vi "Interfacetest.vi"(8 "error in (no error)":errorcluster caption="Fehler (Eingang, kein Fehler)", 11 "Device ID":T1(ring)) -> (0 "error out":errorcluster caption="Fehler (Ausgang)", 3 "Device ID Out":T1(ring))   [LabVIEW 2010]
uses:
  sub VIs v Hauptprogramm/globale Variable 1.vi
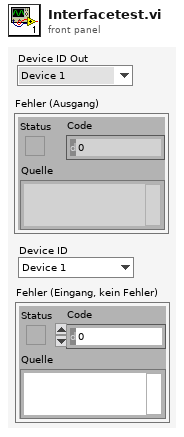
[diagram p1: front panel]
types:
  T1 = enum16{"Device 1", "Device 2", "Device 3", "Device 4", "Device 5", "Device 6", "Device 7", "Device 8"}
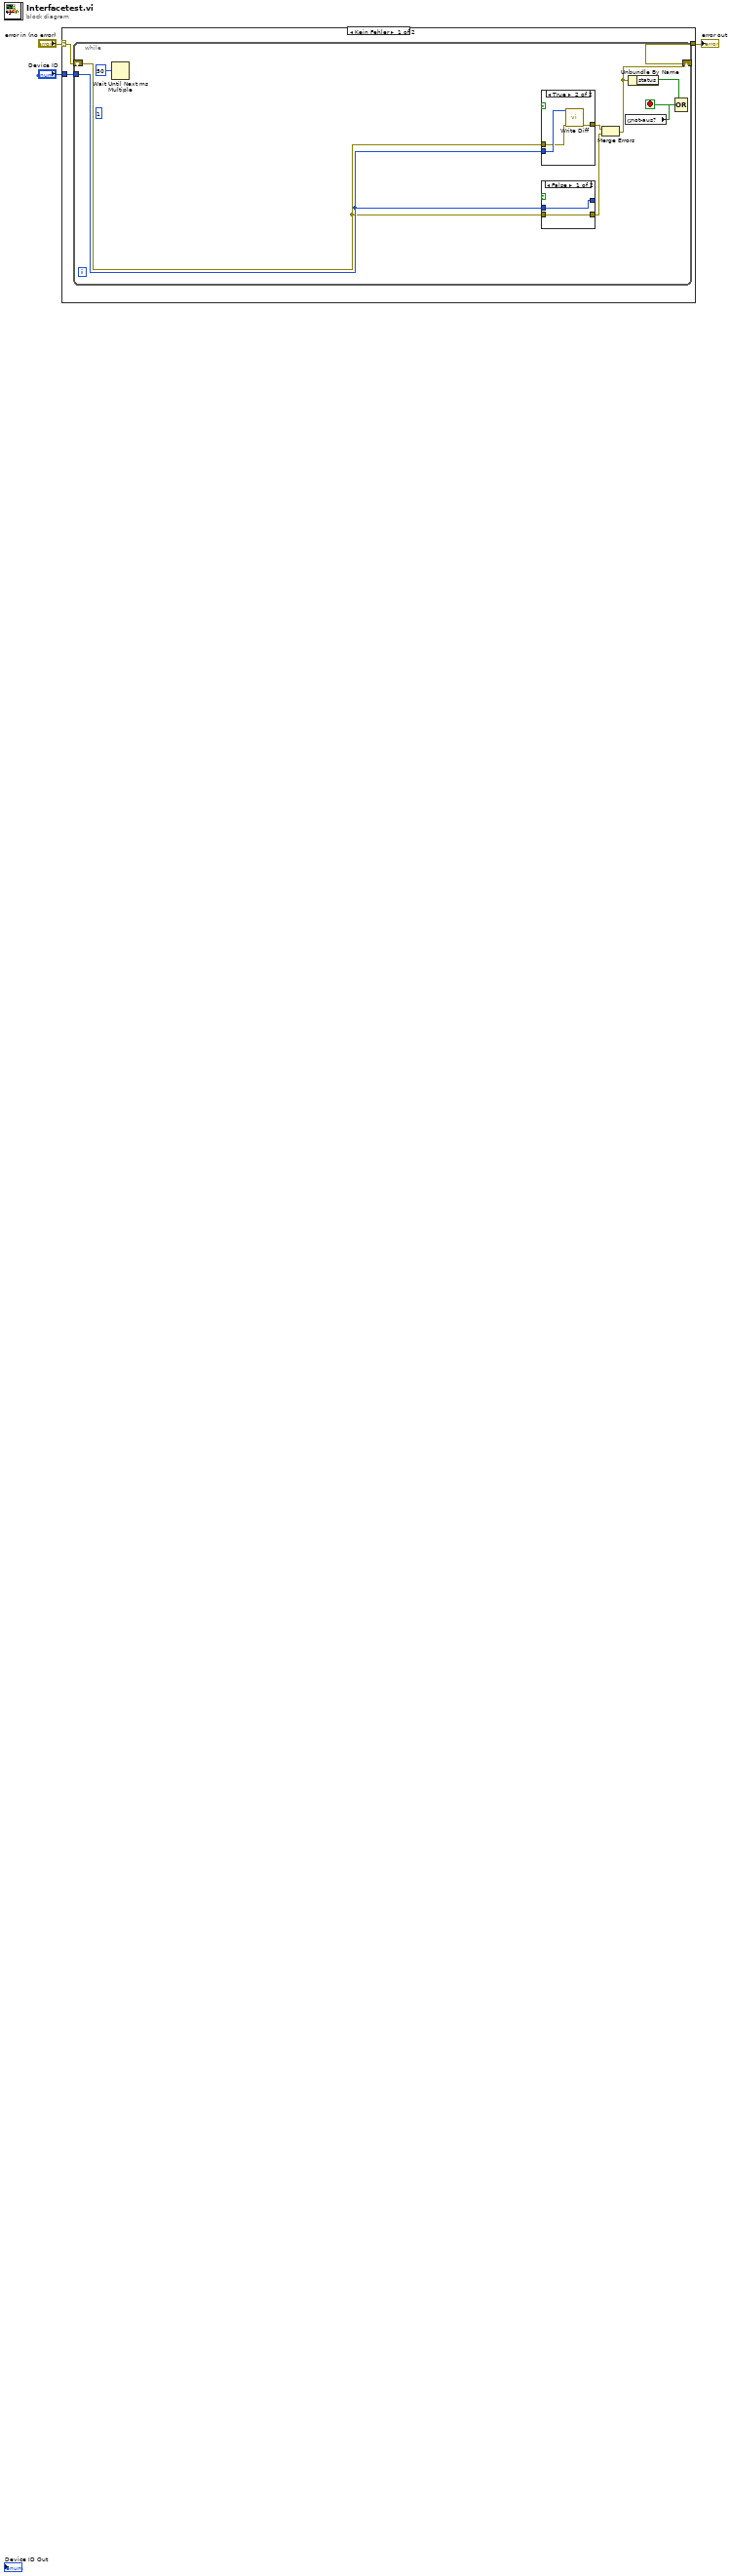
[diagram p0: block diagram]
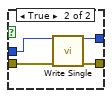
[diagram p3: hidden frame]
diagram:
  n1 = case shown="Kein Fehler" "error in (no error)" {
    selector: "error in (no error)" -> [w5 w26]
    tunnel: [w4 w26] -> w2
    tunnel: "Device ID" -> [w6 _]
    frame No Error {
      n2 = while {
        tunnel: w6 -> [w14]
        shift-right: [w10] -> w4
        shift-left: w5 -> [w11]
        stop <- w7 stop-if-true
        (unwired) 1
        n3 = Wait Until Next ms Multiple(millisecond multiple=50) -> ()  [unwired: 1 out]
        n4 = case shown="True" {
          selector: _ -> [_ _]
          tunnel: w14 -> [_ w19]
          tunnel: [w16 w18] -> w13
          tunnel: w11 -> [w16 w17]
          frame False {
          }
          frame True {
            n5 = call "Write Diff.vi"("Device ID"=w19, "error in"=w17) -> ("error out"=w18:errorcluster)  [unwired: 4 in, 9 out]
          }
        }
        n6 = case shown="False" {
          selector: _ -> [_ _]
          tunnel: [w21 w25] -> _
          tunnel: w14 -> [w21 w24]
          tunnel: [w20 w23] -> w12
          tunnel: w11 -> [w20 w22]
          frame False {
          }
          frame True {
            n7 = call "Write Single.vi"("Device ID"=w24, "error in"=w22) -> ("Device ID Out"=w25:T1, "error out"=w23:errorcluster)  [unwired: 4 in, 8 out]
          }
        }
        n8 = Merge Errors(w13, w12) -> (w10:errorcluster)
        n9 = global read "globale Variable 1.vi" "not-aus?"() -> (w8:bool)
        n10 = Unbundle By Name(w10) -> ("status"=w9:bool)
        n11 = Compound Arithmetic op=OR(w9, w8) -> (w7:bool)  [unwired: 1 in]
      }
    }
    frame Error {
    }
  }
  "error out" <- w2
